vi "Shooting.vi"(6 "Shoot override":dbl, 7 "Serializer Override":dbl, 9 "Lock PWM":bool) -> (0 "Serializer Output":dbl=0.5, 1 "Feeder Output":dbl=1.0, 2 "Shooter \nPWM":dbl=0.7440168132715996, 3 "Rotation Out":dbl=0.09822222222222224)   [LabVIEW 2016]
uses:
  <vilib>/Rock Robotics/Network Tables/NT Read Number.vi
  <vilib>/Rock Robotics/Network Tables/NT Read Numeric Array.vi
  Robot Global Data.vi
  <vilib>/addons/control/pid/pid.llb/PID (DBL).vi
  <vilib>/addons/control/pid/NI_PID_pid.lvlib
panel:
  out "Ball In?":i16(graph)
  out "Image width":dbl(graph)
  out "PWM Output":dbl(graph)
  in  "Lower limit 2":dbl=-3.1 format="%#_13g"
  in  "upper limit 2":dbl=3.1 format="%#_13g"
  out "Object X direct output":dbl(graph)=-7.888888888888889
  out "Object Width":dbl=21.666666666666668
  out "Offset":dbl=5.0 format="%#_13g"
  in  "Lower limit":dbl=-0.1 format="%#_13g"
  in  "upper limit":dbl=0.1 format="%#_13g"
  in  "PID gains":T1={"proportional gain (Kc)"=0.052, "integral time (Ti, min)"=0.0, "derivative time (Td, min)"=0.002} {"derivative time (Td, min)" format="%.3f"; "integral time (Ti, min)" format="%.3f"; "proportional gain (Kc)" format="%.3f"}
  # "Practice Bot\nP: 0.052\nI: 0\nD: 0.002"
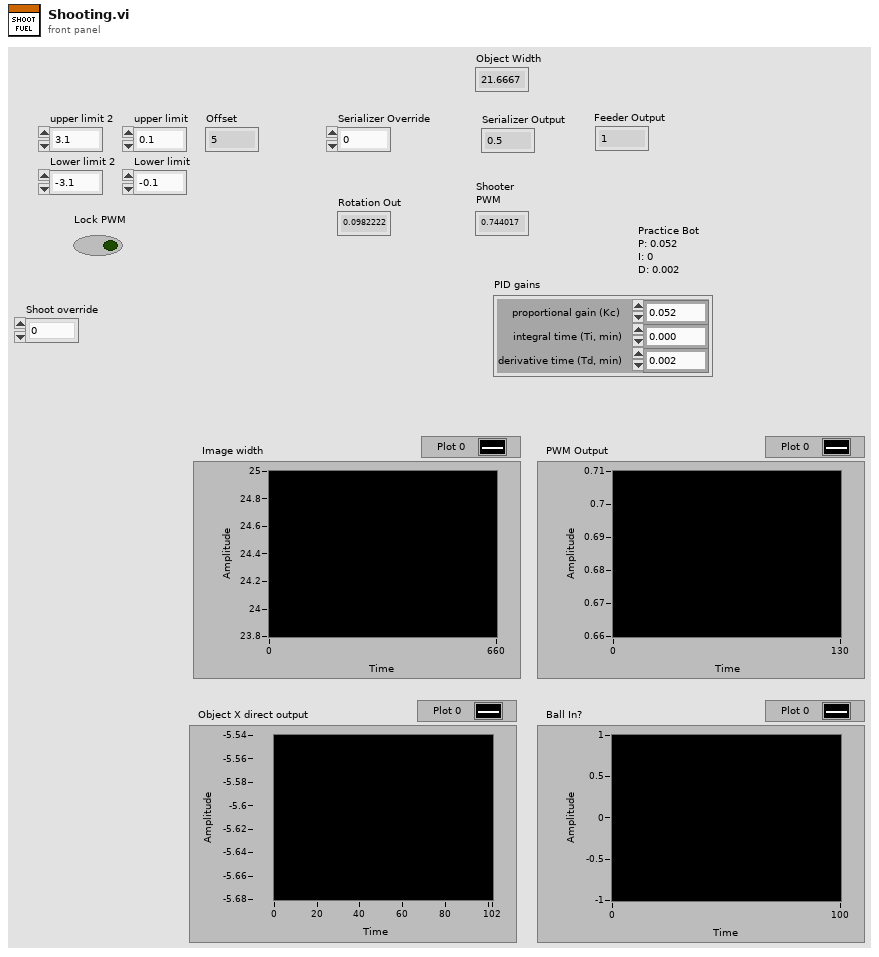
[diagram p1: front panel]
types:
  T1 = cluster{"proportional gain (Kc)":dbl, "integral time (Ti, min)":dbl, "derivative time (Td, min)":dbl}
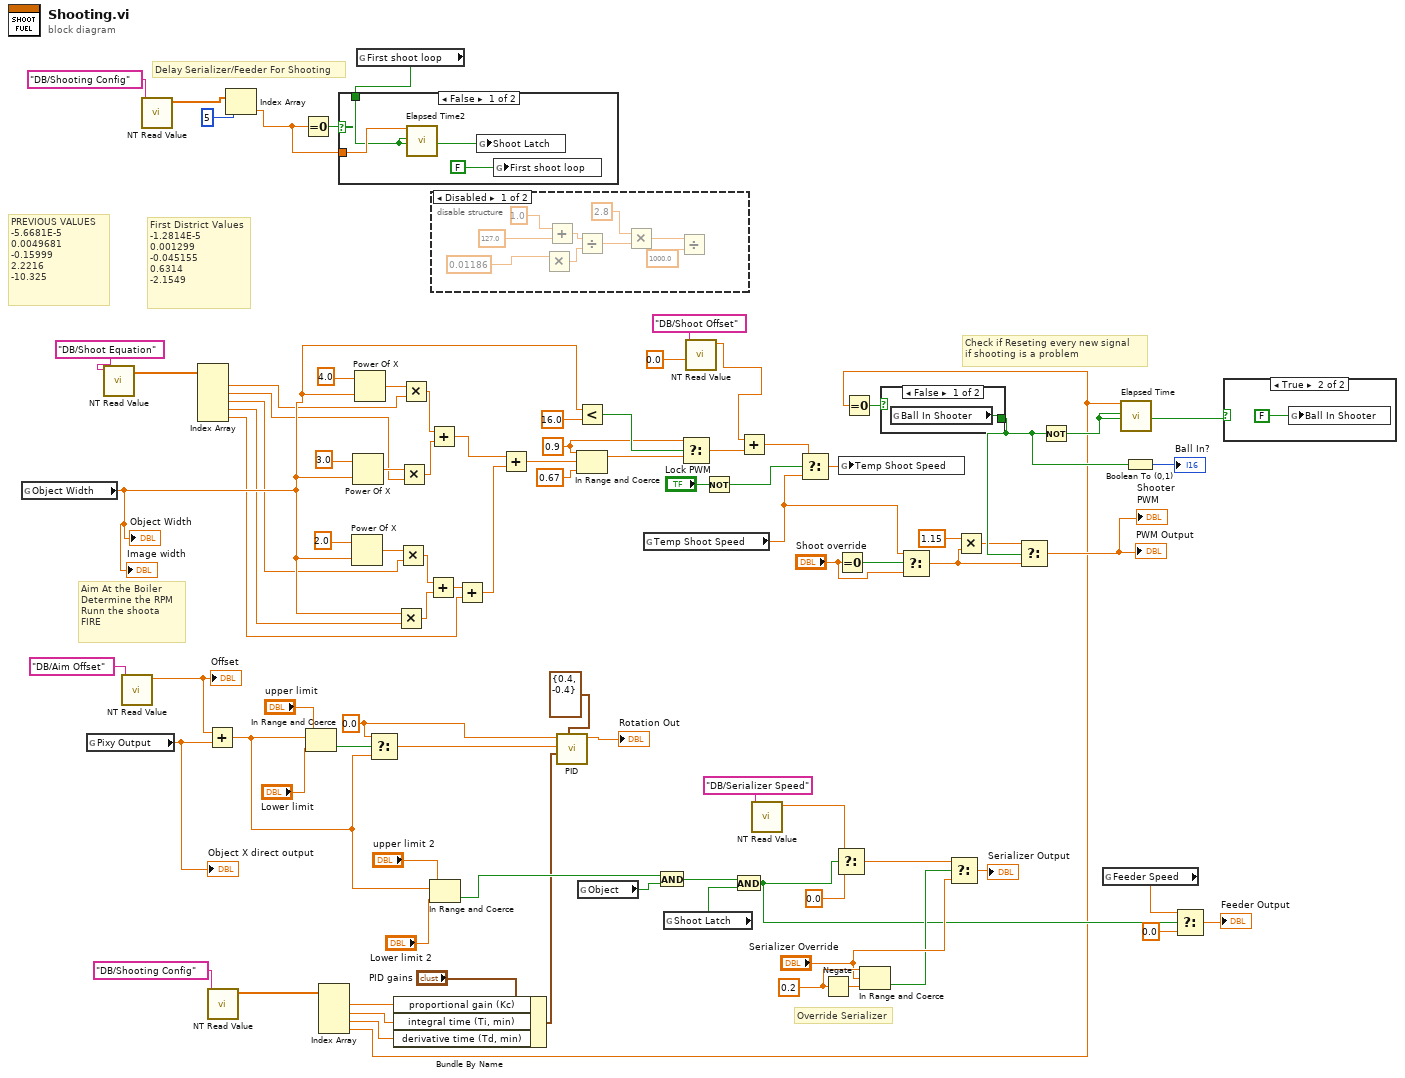
[diagram p0: block diagram]
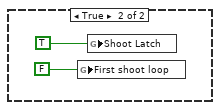
[diagram p2: hidden frame]
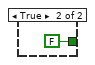
[diagram p3: hidden frame]
diagram:
  w51 = 0.9 ("x")
  w77 = 0.0
  w86 = 0.2
  # "Delay Serializer/Feeder For Shooting"
  # "Check if Reseting every new signal\nif shooting is a problem"
  # "First District Values\n-1.2814E-5\n0.001299\n-0.045155\n0.6314\n-2.1549"
  # "PREVIOUS VALUES\n-5.6681E-5\n0.0049681\n-0.15999\n2.2216\n-10.325"
  # "Override Serializer"
  # "Aim At the Boiler\nDetermine the RPM\nRunn the shoota \nFIRE"
  n1 = global read "Robot Global Data.vi" "Object Width"() -> (w42:dbl)
  "Object Width" <- w42
  "Image width" <- w42
  n2 = global read "Robot Global Data.vi" "Pixy Output"() -> (w61:dbl)
  "Object X direct output" <- w61
  n3 = call-poly <vilib>:"NT Read Value.vi"("Name"="DB/Shoot Equation") -> ("Numeric Array"=w35:dbl[])  [unwired: 9 in, 1 out]
  n4 = call-poly <vilib>:"NT Read Value.vi"("Name"="DB/Aim Offset") -> ("Numeric"=w37:dbl)  [unwired: 9 in, 1 out]
  "Offset" <- w37
  n5 = call-poly <vilib>:"NT Read Value.vi"("Name"="DB/Shooting Config") -> ("Numeric Array"=w4:dbl[])  [unwired: 9 in, 1 out]
  n6 = Index Array(array=w35) -> (element #1=w34:dbl, element #2=w33:dbl, element #3=w32:dbl, element #4=w31:dbl, element #5=w30:dbl)  [unwired: 5 in]
  n7 = Add(x=w37, y=w61) -> (x+y=w57:dbl)
  n8 = call-poly <vilib>:"NT Read Value.vi"("Name"="DB/Shooting Config") -> ("Numeric Array"=w28:dbl[])  [unwired: 9 in, 1 out]
  n9 = Index Array(array=w4, index=5) -> (element=w2:dbl)
  n10 = Equal To 0?(x=w2) -> (x = 0?=w6:bool)
  n11 = In Range and Coerce(upper limit="upper limit", x=w57, lower limit="Lower limit") -> (In Range?=w58:bool)  [unwired: 1 out]
  n12 = Index Array(array=w28) -> (element #1=w26:dbl, element #2=w25:dbl, element #3=w24:dbl, element #4=w7:dbl)  [unwired: 4 in]
  n13 = Power Of X(1:w42, 2:2.0 ("x")) -> (0:w70:dbl)
  n14 = Power Of X(1:w42, 2:3.0 ("x")) -> (0:w72:dbl)
  n15 = Power Of X(1:w42, 2:4.0 ("x")) -> (0:w74:dbl)
  n16 = global read "Robot Global Data.vi" "First shoot loop"() -> (w1:bool)
  n17 = case shown="False" w6 {
    tunnel: w2 -> [w95 _]
    tunnel: w1 -> [w92 _]
    frame False {
      n18 = call "Elapsed Time2"("Time Target (s)"=w95, "Reset"=w92, "Auto Reset"=w92) -> ("Time has Elapsed"=w94:bool)  [unwired: 9 in, 7 out]
      n19 = global write "Robot Global Data.vi" "Shoot Latch"(w94) -> ()
      n20 = global write "Robot Global Data.vi" "First shoot loop"(FALSE ("Time has Elapsed")) -> ()
    }
    frame True {
      n21 = global write "Robot Global Data.vi" "First shoot loop"(FALSE ("Time has Elapsed")) -> ()
      n22 = global write "Robot Global Data.vi" "Shoot Latch"(TRUE ("Time has Elapsed")) -> ()
    }
  }
  n23 = Select(t=w77, s=w58, f=w57) -> (s? t:f=w79:dbl)
  n24 = Bundle By Name(cluster="PID gains", "proportional gain (Kc)"=w26, "integral time (Ti, min)"=w25, "derivative time (Td, min)"=w24) -> (w23:T1)
  n25 = Multiply(x=w42, y=w31) -> (x*y=w66:dbl)
  n26 = Multiply(x=w70, y=w32) -> (x*y=w67:dbl)
  n27 = Multiply(x=w72, y=w33) -> (x*y=w68:dbl)
  n28 = Multiply(x=w74, y=w34) -> (x*y=w69:dbl)
  n29 = Add(x=w67, y=w66) -> (x+y=w65:dbl)
  n30 = Add(x=w69, y=w68) -> (x+y=w63:dbl)
  n31 = In Range and Coerce(upper limit="upper limit 2", x=w57, lower limit="Lower limit 2") -> (In Range?=w56:bool)  [unwired: 1 out]
  n32 = disable-structure shown="Disabled" {
    frame Disabled {
      n33 = Multiply(x=0.01186) -> (x*y=w101:dbl)  [unwired: 1 in]
      n34 = Add(x=1.0, y=127.0) -> (x+y=w105:dbl)
      n35 = Divide(x=w105, y=w101) -> (x/y=w104:dbl)
      n36 = Multiply(x=2.8, y=w104) -> (x*y=w98:dbl)
      n37 = Divide(x=w98, y=1000.0) -> ()  [unwired: 1 out]
    }
    frame Enabled {
    }
  }
  n38 = Add(x=w65, y=w30) -> (x+y=w64:dbl)
  n39 = Add(x=w63, y=w64) -> (x+y=w54:dbl)
  n40 = call-poly <vilib>:"PID.vi"("output range"=cluster{"output high":dbl, "output low":dbl} {"output high"=0.4, "output low"=-0.4}, "PID gains"=w23, "process variable"=w79, "setpoint"=w77) -> ("output"=→"Rotation Out":dbl)  [unwired: 6 in, 1 out]
  n41 = Less?(x=w42, y=16.0) -> (x < y?=w53:bool)
  n42 = In Range and Coerce(upper limit=w51, x=w54, lower limit=0.67 ("x")) -> (coerced(x)=w52:dbl)  [unwired: 1 out]
  n43 = global read "Robot Global Data.vi" "Object"() -> (w47:bool)
  n44 = global read "Robot Global Data.vi" "Temp Shoot Speed"() -> (w40:dbl)
  n45 = And(x=w56, y=w47) -> (x .and. y?=w19:bool)
  n46 = global read "Robot Global Data.vi" "Shoot Latch"() -> (w18:bool)
  n47 = Select(t=w51, s=w53, f=w52) -> (s? t:f=w50:dbl)
  n48 = call-poly <vilib>:"NT Read Value.vi"("Default Value"=0.0, "Name"="DB/Shoot Offset") -> ("Numeric"=w44:dbl)  [unwired: 8 in, 1 out]
  n49 = Not(x="Lock PWM") -> (.not. x?=w49:bool)
  n50 = And(x=w19, y=w18) -> (x .and. y?=w17:bool)
  n51 = Add(x=w44, y=w50) -> (x+y=w46:dbl)
  n52 = call-poly <vilib>:"NT Read Value.vi"("Name"="DB/Serializer Speed") -> ("Numeric"=w90:dbl)  [unwired: 9 in, 1 out]
  n53 = Select(t=w46, s=w49, f=w40) -> (s? t:f=w78:dbl)
  n54 = Negate(x=w86) -> (-x=w87:dbl)
  n55 = Select(t=w90, s=w17, f=0.0) -> (s? t:f=w85:dbl)
  n56 = Equal To 0?(x="Shoot override") -> (x = 0?=w41:bool)
  n57 = global write "Robot Global Data.vi" "Temp Shoot Speed"(w78) -> ()
  n58 = Equal To 0?(x=w7) -> (x = 0?=w8:bool)
  n59 = In Range and Coerce(upper limit=w86, x="Serializer Override", lower limit=w87) -> (In Range?=w76:bool)  [unwired: 1 out]
  n60 = case shown="False" w8 {
    tunnel: [w107 FALSE ("Ball In Shooter")] -> w13
    frame False {
      n61 = global read "Robot Global Data.vi" "Ball In Shooter"() -> (w107:bool)
    }
    frame True {
    }
  }
  n62 = Select(t=w40, s=w41, f="Shoot override") -> (s? t:f=w9:dbl)
  n63 = Select(t=w85, s=w76, f="Serializer Override") -> (s? t:f=→"Serializer Output":dbl)
  n64 = Multiply(x=1.15 ("t"), y=w9) -> (x*y=w10:dbl)
  n65 = Select(t=w10, s=w13, f=w9) -> (s? t:f=→"Shooter \nPWM" →"PWM Output":dbl)
  n66 = Not(x=w13) -> (.not. x?=w20:bool)
  n67 = global read "Robot Global Data.vi" "Feeder Speed"() -> (w15:dbl)
  n68 = call "Elapsed Time"("Time Target (s)"=w7, "Reset"=w20, "Auto Reset"=w20) -> ("Time has Elapsed"=w21:bool)  [unwired: 9 in, 7 out]
  n69 = Boolean To (0,1)(Boolean=w13) -> (0, 1=→"Ball In?":i16)
  n70 = Select(t=w15, s=w17, f=0.0) -> (s? t:f=→"Feeder Output":dbl)
  n71 = case shown="True" w21 {
    frame False {
    }
    frame True {
      n72 = global write "Robot Global Data.vi" "Ball In Shooter"(FALSE) -> ()
    }
  }
